vi "Accumulate Data.vi"(8 "Error in":errorcluster, 10 "New Data":dbl[](array[numeric]), 11 "State Variables in":T1={"Stop Notifier"=refnum, "UI References"=[], "DAQmx"={"ECG Input"={"Channel"="", "Task"="", "Max Value"=0.0, "Min Value"=0.0, "Sampling Rate"=0.0, "Batch Size"=10}, "Trigger Output"={"Channel"="", "Task"="", "Pulse Frequency"=0.0, "Delay"=0, "Triggers per Shot"=0}}, "Data Queue"=refnum, "Filter"={"Batch Size"=1000, "Update Cycle"=0, "Filter Buffer"=[]}, "Last Detect Result"=FALSE}) -> (0 "Error out":errorcluster, 2 "Buffered Data":dbl[](array[numeric]), 3 "State Variables out":T1={"Stop Notifier"=refnum, "UI References"=[], "DAQmx"={"ECG Input"={"Channel"="", "Task"="", "Max Value"=0.0, "Min Value"=0.0, "Sampling Rate"=0.0, "Batch Size"=10}, "Trigger Output"={"Channel"="", "Task"="", "Pulse Frequency"=0.0, "Delay"=0, "Triggers per Shot"=0}}, "Data Queue"=refnum, "Filter"={"Batch Size"=1000, "Update Cycle"=0, "Filter Buffer"=[]}, "Last Detect Result"=FALSE}, 5 "Is Buffer Ready?":bool)   [LabVIEW 2014, in "Filter.lvlib"]
uses:
  Filter.lvlib
  Controls/State Variables.ctl
  Controls/DAQmx Variables.ctl
  Controls/Filter Variables.ctl
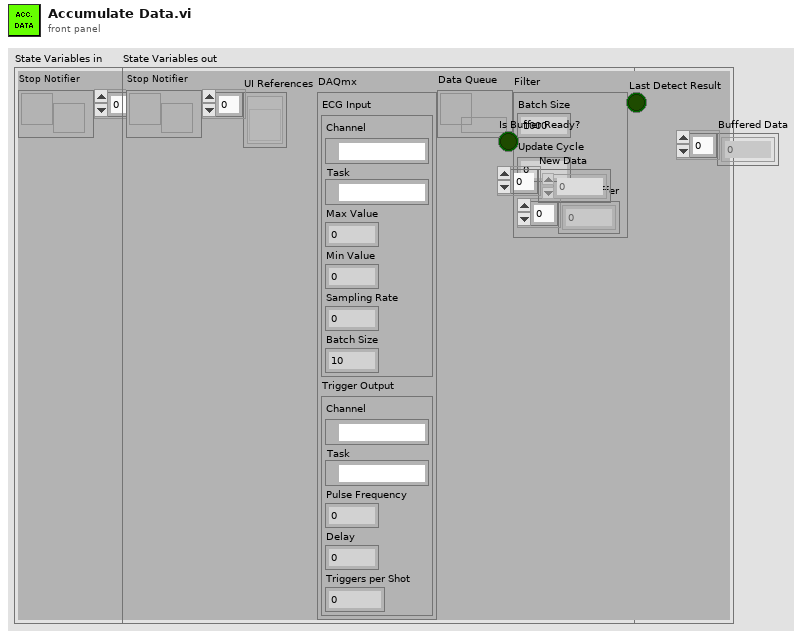
[diagram p1: front panel]
types:
  T1 = typedef "State Variables.ctl" = cluster{"Stop Notifier":refnum<notifier>, "UI References":refnum<vi>[], "DAQmx":T2, "Data Queue":refnum<queue>, "Filter":T3, "Last Detect Result":bool}
  T2 = typedef "DAQmx Variables.ctl" = cluster{"ECG Input":cluster{"Channel":tag, "Task":refnum<k21>, "Max Value":dbl, "Min Value":dbl, "Sampling Rate":dbl, "Batch Size":i32}, "Trigger Output":cluster{"Channel":tag, "Task":refnum<k21>, "Pulse Frequency":dbl, "Delay":u16, "Triggers per Shot":i32}}
  T3 = typedef "Filter Variables.ctl" = cluster{"Batch Size":i32, "Update Cycle":i32, "Filter Buffer":dbl[]}
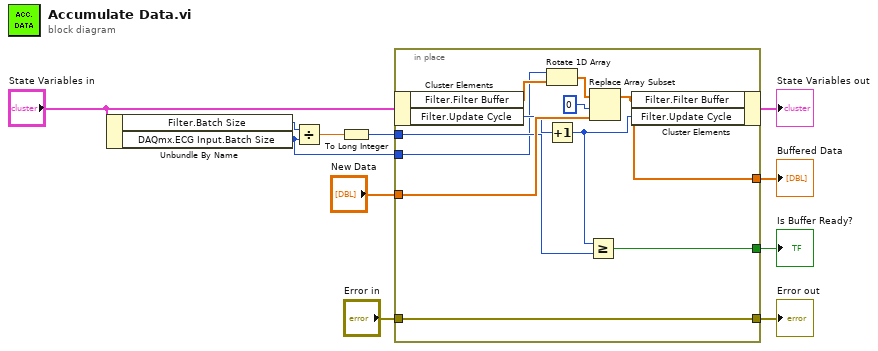
[diagram p0: block diagram]
diagram:
  n1 = Unbundle By Name("State Variables in") -> ("Filter.Batch Size"=w4:i32, "DAQmx.ECG Input.Batch Size"=w1:i32)
  n2 = Divide(x=w4, y=w1) -> (x/y=w3:dbl)
  n3 = To Long Integer(number=w3) -> (32bit integer=w2:i32)
  n4 = in-place {
    in-place-border: "New Data" -> [w19]
    in-place-border: [w18] -> w10
    in-place-border: "Error in" -> [w18]
    in-place-border: [w17] -> w7
    in-place-border: [w14] -> w5
    in-place-border: w2 -> [w13]
    in-place-border: w1 -> [w12]
    n5 = in-place-cluster #1("State Variables in") -> ("Filter.Filter Buffer"=w20:dbl[], "Filter.Update Cycle"=w16:i32)
    n6 = Rotate 1D Array(1:w20, 2:w12) -> (0:w21:dbl[])
    n7 = Increment(x=w16) -> (x+1=w15:i32)
    n8 = Greater Or Equal?(x=w15, y=w13) -> (x >= y?=w14:bool)
    n9 = Replace Array Subset(array=w21, new element=w19, index=0) -> (w17:dbl[])
    n10 = in-place-cluster #1("Filter.Filter Buffer"=w17, "Filter.Update Cycle"=w15) -> (→"State Variables out":T1)
  }
  "Error out" <- w10
  "Is Buffer Ready?" <- w5
  "Buffered Data" <- w7
